vi "Build Command.vi"(0 "Database":string, 1 "Database Command":T1, 2 "Query":bool, 5 "Table":string, 7 "Column List":string[](array[string]), 9 "Values":string[](array[string]), 11 "error in (no error)":errorcluster, 12 "Condition":string, 13 "SQL Command in":string) -> (4 "SQL Command out":string, 6 "Query?":bool, 15 "error out":errorcluster)   [LabVIEW 2017, in "VIs to Interface LabVIEW and MySQL dotNET Connector.lvlib"]
doc: "This VI encapsulates common SQL commands and provides the formatting to go from LabVIEW data to SQL command."
uses:
  VIs to Interface LabVIEW and MySQL dotNET Connector.lvlib
  Controls/Database Command.ctl
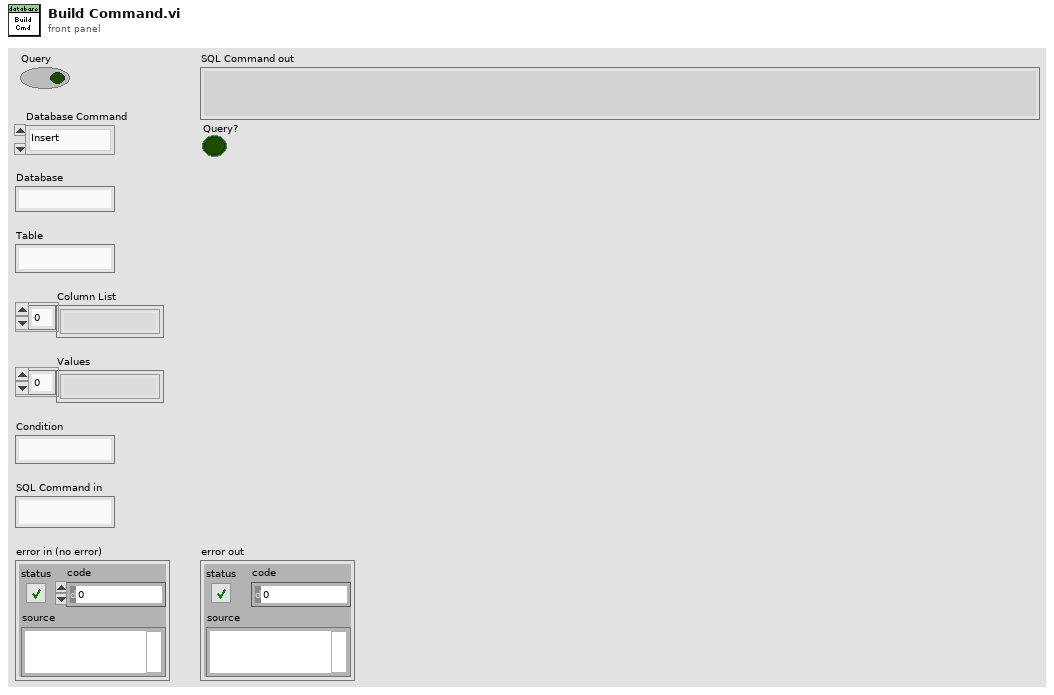
[diagram p1: front panel]
types:
  T1 = typedef "VIs to Interface LabVIEW and MySQL dotNET Connector.lvlib/Database Command.ctl" = enum16{"Insert", "Update", "Select All", "Delete Entry", "Drop Table", "SQL Command", "Select", "Get Column Info", "Select Column"}
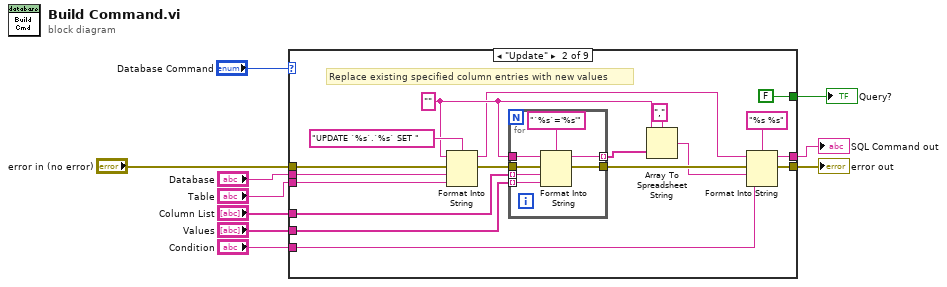
[diagram p0: block diagram]
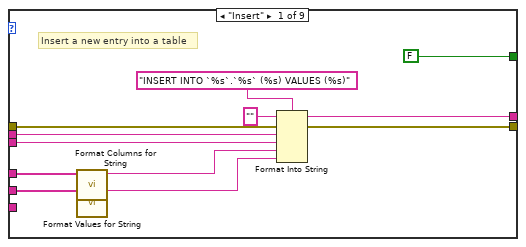
[diagram p2: hidden frame]
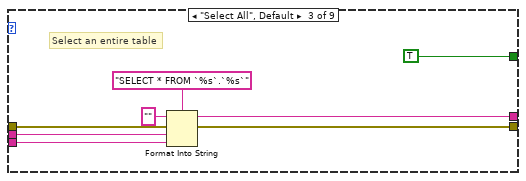
[diagram p3: hidden frame]
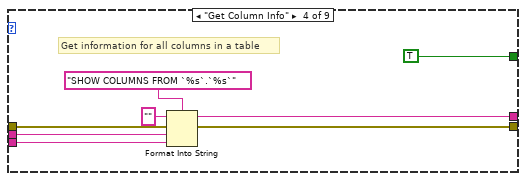
[diagram p4: hidden frame]
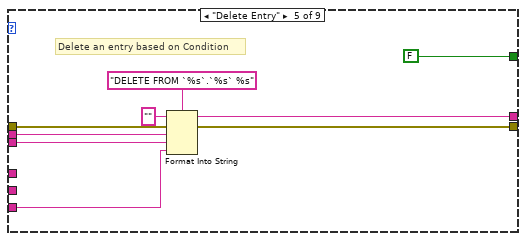
[diagram p5: hidden frame]
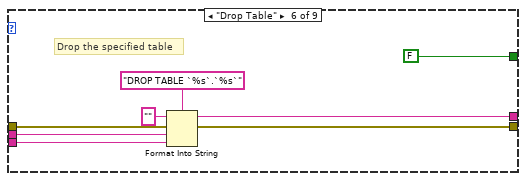
[diagram p6: hidden frame]
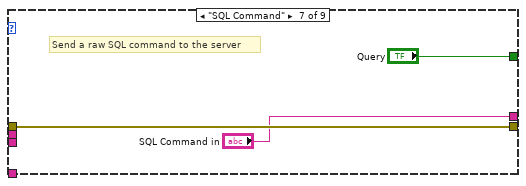
[diagram p7: hidden frame]
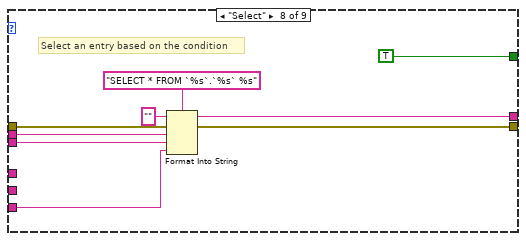
[diagram p8: hidden frame]
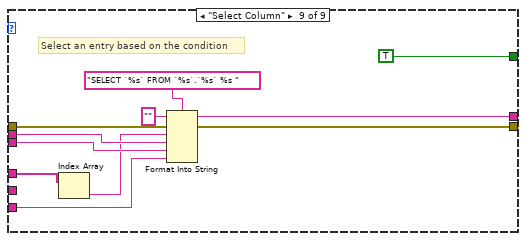
[diagram p9: hidden frame]
diagram:
  n1 = case shown="\"Update\"" "Database Command" {
    tunnel: "Database" -> [w20 w38 w53 w61 w70 w78 _ w90 w95]
    tunnel: "Table" -> [w19 w37 w52 w60 w69 w77 _ w89 w101]
    tunnel: "Column List" -> [w17 w36 _ _ _ _ _ _ w96]
    tunnel: "Values" -> [w16 w35 _ _ _ _ _ _ _]
    tunnel: [w12 w32 w50 w58 w67 w75 "SQL Command in" w87 w99] -> w10
    tunnel: [w13 w31 w49 w57 w66 w74 w83 w86 w98] -> w9
    tunnel: "error in (no error)" -> [w18 w30 w51 w59 w68 w76 w83 w88 w100]
    tunnel: "Condition" -> [_ w26 _ _ w65 _ _ w85 w93]
    tunnel: [FALSE FALSE TRUE TRUE FALSE FALSE "Query" TRUE TRUE] -> w1
    frame "Insert" {
      # "Insert a new entry into a table"
      n2 = call "Format Columns for String.vi"("Column List"=w17) -> ("Column String"=w15:string)  [unwired: 10 in]
      n3 = call "Format Values for String.vi"("Values"=w16) -> ("Value String"=w14:string)  [unwired: 10 in]
      n4 = Format Into String(format string="INSERT INTO `%s`.`%s` (%s) VALUES (%s)", initial string="", error in=w18, w20, w19, w15, w14) -> (resulting string=w12:string, error out=w13:errorcluster)
    }
    frame "Update" {
      w24 = "" ("initial string")
      # "Replace existing specified column entries with new values"
      n5 = Format Into String(format string="UPDATE `%s`.`%s` SET ", initial string=w24, error in=w30, w38, w37) -> (resulting string=w23:string, error out=w39:errorcluster)
      n6 = for {
        tunnel: w39 -> [w47]
        tunnel: [w44] -> w34
        tunnel: w36 -> [w43] mode=indexing
        tunnel: w35 -> [w42] mode=indexing
        tunnel: [w45] -> w28 mode=indexing
        tunnel: w24 -> [w41]
        n7 = Format Into String(format string="`%s`='%s'", initial string=w41, error in=w47, w43, w42) -> (resulting string=w45:string, error out=w44:errorcluster)
      }
      n8 = Array To Spreadsheet String(delimiter (Tab)=",", array=w28, 3:w24) -> (spreadsheet string=w25:string)
      n9 = Format Into String(format string="%s %s", initial string=w23, error in=w34, w25, w26) -> (resulting string=w32:string, error out=w31:errorcluster)
    }
    frame "Select All", Default {
      # "Select an entire table"
      n10 = Format Into String(format string="SELECT * FROM `%s`.`%s`", initial string="", error in=w51, w53, w52) -> (resulting string=w50:string, error out=w49:errorcluster)
    }
    frame "Get Column Info" {
      # "Get information for all columns in a table"
      n11 = Format Into String(format string="SHOW COLUMNS FROM `%s`.`%s`", initial string="", error in=w59, w61, w60) -> (resulting string=w58:string, error out=w57:errorcluster)
    }
    frame "Delete Entry" {
      # "Delete an entry based on Condition"
      n12 = Format Into String(format string="DELETE FROM `%s`.`%s` %s", initial string="", error in=w68, w70, w69, w65) -> (resulting string=w67:string, error out=w66:errorcluster)
    }
    frame "Drop Table" {
      # "Drop the specified table"
      n13 = Format Into String(format string="DROP TABLE `%s`.`%s`", initial string="", error in=w76, w78, w77) -> (resulting string=w75:string, error out=w74:errorcluster)
    }
    frame "SQL Command" {
      # "Send a raw SQL command to the server"
    }
    frame "Select" {
      # "Select an entry based on the condition"
      n14 = Format Into String(format string="SELECT * FROM `%s`.`%s` %s", initial string="", error in=w88, w90, w89, w85) -> (resulting string=w87:string, error out=w86:errorcluster)
    }
    frame "Select Column" {
      # "Select an entry based on the condition"
      n15 = Index Array(array=w96) -> (element=w94:string)  [unwired: 1 in]
      n16 = Format Into String(format string="SELECT `%s` FROM `%s`.`%s` %s ", initial string="", error in=w100, w94, w95, w101, w93) -> (resulting string=w99:string, error out=w98:errorcluster)
    }
  }
  "SQL Command out" <- w10
  "error out" <- w9
  "Query?" <- w1
